vi "ma_sml_M-1 Decimator with IC.vi"   [LabVIEW 2020, in "NI_MAPro.lvlib"]
uses:
  NI_MAPro.lvlib
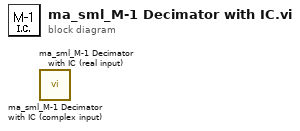
[diagram p0: block diagram]
diagram:
  n1 = call "ma_sml_M-1 Decimator with IC (complex input).vi"() -> ()  [unwired: 5 in, 2 out]
  n2 = call "ma_sml_M-1 Decimator with IC (real input).vi"() -> ()  [unwired: 5 in, 2 out]
